vi "Update_Rem_gas.vi"(2 "Scan Period (s)":dbl format="%.2f", 4 "Gas Remaining in":dbl format="%.3f", 5 "Ch name":string, 6 "Ch names":string[](array[string]), 7 "Present scan array":dbl[](array[numeric]) format="%.2f") -> (0 "Gas Remaining out":dbl format="%.3f", 1 "Comments":string)   [LabVIEW 2020]
uses:
  Anemometry/Anemometry Sub Vis/Globals/Gas_management_global.vi
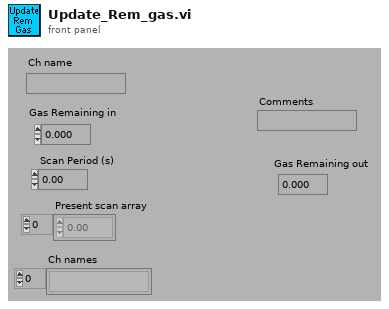
[diagram p1: front panel]
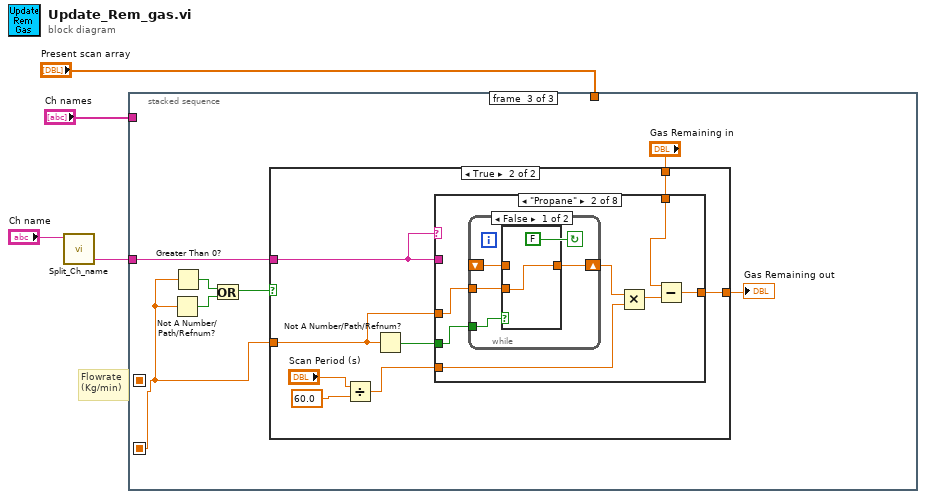
[diagram p0: block diagram]
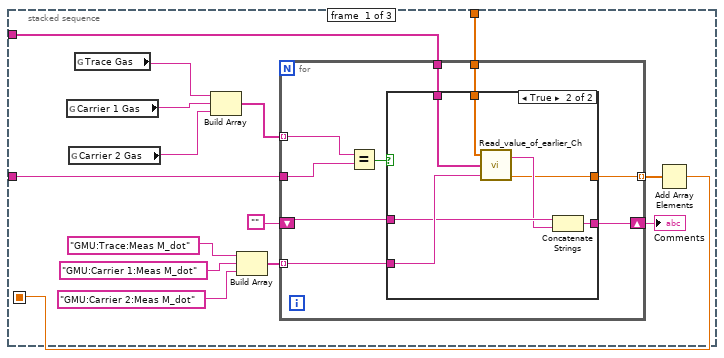
[diagram p2: hidden frame]
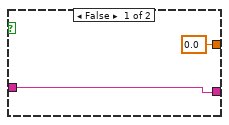
[diagram p3: hidden frame]
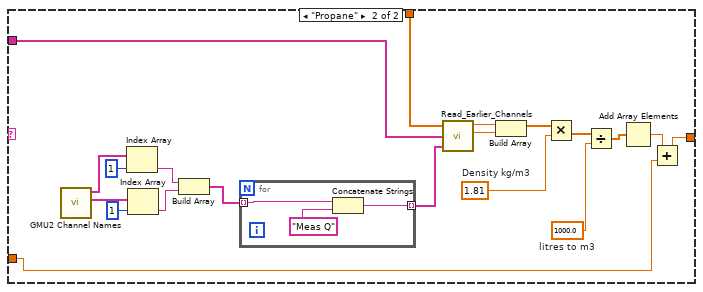
[diagram p5: hidden frame]
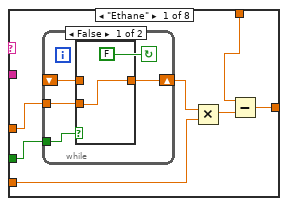
[diagram p7: hidden frame]
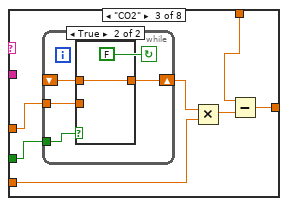
[diagram p10: hidden frame]
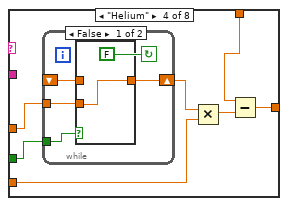
[diagram p12: hidden frame]
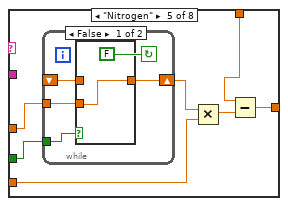
[diagram p14: hidden frame]
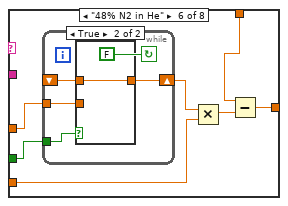
[diagram p16: hidden frame]
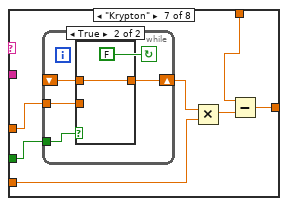
[diagram p18: hidden frame]
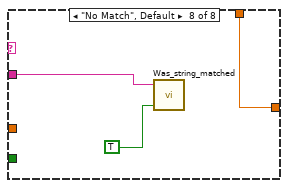
[diagram p20: hidden frame]
diagram:
  # "Flowrate\n(Kg/min)"
  n1 = call "Split_Ch_name.vi"("Ch name"="Ch name") -> ("Low level"=w3:string)  [unwired: 2 out]
  n2 = stacked-sequence {
    seq-local: [w11 _ _] -> [_ w38 _]
    seq-local: [_ w39 _] -> [_ _ w67]
    tunnel: w3 -> [w14 w42 w71]
    tunnel: "Present scan array" -> [w6 w41 _]
    tunnel: "Ch names" -> [w5 w40 _]
    frame #0 {
      n3 = global read "Gas_management_global.vi" "Carrier 1 Gas"() -> (w19:string)
      n4 = global read "Gas_management_global.vi" "Carrier 2 Gas"() -> (w8:string)
      n5 = global read "Gas_management_global.vi" "Trace Gas"() -> (w18:string)
      n6 = Build Array(w18, w19, w8) -> (w15:string[])
      n7 = Build Array("GMU:Trace:Meas M_dot" ("Desired Ch to Read"), "GMU:Carrier 1:Meas M_dot" ("Desired Ch to Read"), "GMU:Carrier 2:Meas M_dot" ("Desired Ch to Read")) -> (w13:string[])
      n8 = for {
        tunnel: w15 -> [w22] mode=indexing
        tunnel: w14 -> [w28]
        tunnel: w13 -> [w26] mode=indexing
        shift-right: [w24] -> w10
        shift-left: "" -> [w25]
        tunnel: [w23] -> w12 mode=indexing
        tunnel: w6 -> [w21]
        tunnel: w5 -> [w20]
        n9 = Equal?(x=w22, y=w28) -> (x = y?=w27:bool)
        n10 = case shown="True" w27 {
          tunnel: w26 -> [_ w37]
          tunnel: w25 -> [w29 w36]
          tunnel: [w29 w34] -> w24
          tunnel: [0.0 ("Value") w33] -> w23
          tunnel: w21 -> [_ w32]
          tunnel: w20 -> [_ w31]
          frame False {
          }
          frame True {
            n11 = call "Read_value_of_earlier_Ch.vi"("Desired Ch to Read"=w37, "Ch names"=w31, "Present scan array"=w32) -> ("Value"=w33:dbl, "Scan comment"=w35:string)  [unwired: 1 in]
            n12 = Concatenate Strings(w36, w35) -> (w34:string)
          }
        }
      }
      "Comments" <- w10
      n13 = Add Array Elements(numeric array=w12) -> (sum=w11:dbl)
    }
    frame #1 {
      n14 = case shown="Default" w42 {
        tunnel: w41 -> [_ w56]
        tunnel: w40 -> [_ w55]
        tunnel: [w43 w45] -> w39
        tunnel: w38 -> [w43 w44]
        frame Default {
        }
        frame "Propane" {
          w48 = 1000.0  # litres to m3
          w50 = 1.81  # Density kg/m3
          n15 = call "GMU2 Channel Names.vi"() -> ("GMU2 Source Channels"=w62:string[], "GMU2 Calib Channels"=w63:string[])  [unwired: 10 in]
          n16 = Index Array(array=w63, index=1) -> (element=w58:string)
          n17 = Index Array(array=w62, index=1) -> (element=w59:string)
          n18 = Build Array(w58, w59) -> (w57:string[])
          n19 = for {
            tunnel: w57 -> [w65] mode=indexing
            tunnel: [w64] -> w54 mode=indexing
            n20 = Concatenate Strings(w65, "Meas Q" ("string")) -> (w64:string)
          }
          n21 = call "Read_Earlier_Channels.vi"("Present scan array"=w56, "Ch names"=w55, "Desired Channels"=w54) -> ("Index 0"=w53:dbl, "Index 1"=w52:dbl)  [unwired: 4 out]
          n22 = Build Array(w53, w52) -> (w51:dbl[])
          n23 = Multiply(x=w51, y=w50) -> (x*y=w49:dbl[])
          n24 = Divide(x=w49, y=w48) -> (x/y=w47:dbl[])
          n25 = Add Array Elements(numeric array=w47) -> (sum=w46:dbl)
          n26 = Add(x=w46, y=w44) -> (x+y=w45:dbl)
        }
      }
    }
    frame #2 {
      n27 = Not A Number/Path/Refnum?(number/path/refnum=w67) -> (NaN/Path/Refnum?=w70:bool)
      n28 = Greater Than 0?(x=w67) -> (x > 0?=w69:bool)
      n29 = Or(x=w69, y=w70) -> (x .or. y?=w68:bool)
      n30 = case shown="True" w68 {
        tunnel: [w74 w79] -> w73
        tunnel: "Gas Remaining in" -> [w74 w78]
        tunnel: w67 -> [_ w76]
        tunnel: w71 -> [_ w75]
        frame False {
        }
        frame True {
          n31 = Divide(x="Scan Period (s)", y=60.0) -> (x/y=w82:dbl)
          n32 = Not A Number/Path/Refnum?(number/path/refnum=w76) -> (NaN/Path/Refnum?=w77:bool)
          n33 = case shown="\"Propane\"" w75 {
            tunnel: w77 -> [w88 w102 w116 w130 w144 w158 w172 _]
            tunnel: w76 -> [w89 w103 w117 w131 w145 w159 w173 _]
            tunnel: w82 -> [w86 w100 w114 w128 w142 w156 w170 _]
            tunnel: [w84 w98 w112 w126 w140 w153 w167 w183] -> w79
            tunnel: w78 -> [w83 w97 w111 w125 w139 w154 w168 w183]
            tunnel: w75 -> [_ _ _ _ _ _ _ w182]
            frame "Ethane" {
              n34 = while {
                tunnel: w89 -> [w91]
                tunnel: w88 -> [w94]
                shift-left: _ -> [w92]
                shift-right: [w93] -> w85
                stop <- FALSE continue-if-true
                n35 = case shown="False" w94 {
                  tunnel: [w95 w96] -> w93
                  tunnel: w92 -> [_ w96]
                  tunnel: w91 -> [w95 _]
                  frame False {
                  }
                  frame True {
                  }
                }
              }
              n36 = Multiply(x=w85, y=w86) -> (x*y=w87:dbl)
              n37 = Subtract(x=w83, y=w87) -> (x-y=w84:dbl)
            }
            frame "Propane" {
              n38 = while {
                tunnel: w103 -> [w105]
                tunnel: w102 -> [w108]
                shift-left: _ -> [w106]
                shift-right: [w107] -> w99
                stop <- FALSE continue-if-true
                n39 = case shown="False" w108 {
                  tunnel: [w109 w110] -> w107
                  tunnel: w106 -> [_ w110]
                  tunnel: w105 -> [w109 _]
                  frame False {
                  }
                  frame True {
                  }
                }
              }
              n40 = Multiply(x=w99, y=w100) -> (x*y=w101:dbl)
              n41 = Subtract(x=w97, y=w101) -> (x-y=w98:dbl)
            }
            frame "CO2" {
              n42 = while {
                tunnel: w117 -> [w119]
                tunnel: w116 -> [w122]
                shift-left: _ -> [w120]
                shift-right: [w121] -> w113
                stop <- FALSE continue-if-true
                n43 = case shown="True" w122 {
                  tunnel: [w123 w124] -> w121
                  tunnel: w120 -> [_ w124]
                  tunnel: w119 -> [w123 _]
                  frame False {
                  }
                  frame True {
                  }
                }
              }
              n44 = Multiply(x=w113, y=w114) -> (x*y=w115:dbl)
              n45 = Subtract(x=w111, y=w115) -> (x-y=w112:dbl)
            }
            frame "Helium" {
              n46 = while {
                tunnel: w131 -> [w133]
                tunnel: w130 -> [w136]
                shift-left: _ -> [w134]
                shift-right: [w135] -> w127
                stop <- FALSE continue-if-true
                n47 = case shown="False" w136 {
                  tunnel: [w137 w138] -> w135
                  tunnel: w134 -> [_ w138]
                  tunnel: w133 -> [w137 _]
                  frame False {
                  }
                  frame True {
                  }
                }
              }
              n48 = Multiply(x=w127, y=w128) -> (x*y=w129:dbl)
              n49 = Subtract(x=w125, y=w129) -> (x-y=w126:dbl)
            }
            frame "Nitrogen" {
              n50 = while {
                tunnel: w145 -> [w147]
                tunnel: w144 -> [w150]
                shift-left: _ -> [w148]
                shift-right: [w149] -> w141
                stop <- FALSE continue-if-true
                n51 = case shown="False" w150 {
                  tunnel: [w151 w152] -> w149
                  tunnel: w148 -> [_ w152]
                  tunnel: w147 -> [w151 _]
                  frame False {
                  }
                  frame True {
                  }
                }
              }
              n52 = Multiply(x=w141, y=w142) -> (x*y=w143:dbl)
              n53 = Subtract(x=w139, y=w143) -> (x-y=w140:dbl)
            }
            frame "48% N2 in He" {
              n54 = while {
                tunnel: w159 -> [w161]
                tunnel: w158 -> [w164]
                shift-left: _ -> [w162]
                shift-right: [w163] -> w155
                stop <- FALSE continue-if-true
                n55 = case shown="True" w164 {
                  tunnel: [w165 w166] -> w163
                  tunnel: w162 -> [_ w166]
                  tunnel: w161 -> [w165 _]
                  frame False {
                  }
                  frame True {
                  }
                }
              }
              n56 = Multiply(x=w155, y=w156) -> (x*y=w157:dbl)
              n57 = Subtract(x=w154, y=w157) -> (x-y=w153:dbl)
            }
            frame "Krypton" {
              n58 = while {
                tunnel: w173 -> [w175]
                tunnel: w172 -> [w178]
                shift-left: _ -> [w176]
                shift-right: [w177] -> w169
                stop <- FALSE continue-if-true
                n59 = case shown="True" w178 {
                  tunnel: [w179 w180] -> w177
                  tunnel: w176 -> [_ w180]
                  tunnel: w175 -> [w179 _]
                  frame False {
                  }
                  frame True {
                  }
                }
              }
              n60 = Multiply(x=w169, y=w170) -> (x*y=w171:dbl)
              n61 = Subtract(x=w168, y=w171) -> (x-y=w167:dbl)
            }
            frame "No Match", Default {
              n62 = call "Was_string_matched.vi"("Match Error"=TRUE, "Variable name"=w182) -> ()  [unwired: 1 in]
            }
          }
        }
      }
      "Gas Remaining out" <- w73
    }
  }
